vi "TEST_L0_MAJnADDS_NEW.vi"(0 "Instrument VISA in":T1={"AWG VISA"="generadorpulsos", "Oscilloscope  VISA "="Oscilloscope", "Integration Board IP"="172.16.7.43", "connection ID"=refnum, "report out"=refnum, "report file path"=path "C:/Documents and Settings/CTA_LAB01/Desktop/L0_Asic/L0 Asic Test Data"}, 1 "threshold":i32[][](array[numeric])=[[518, 513, 533, 498, 543, 508, 548], [526, 521, 546, 506, 551, 516, 556], [534, 529, 549, 514, 559, 524, 564], [542, 537, 557, 522, 567, 532, 572], [545, 540, 565, 530, 575, 530, 575]], 2 "Serial number":string="SN_023", 11 "error in":errorcluster, 13 "Voltages comprobation":dbl[](array[numeric])=[0.05, 0.1, 0.2, 0.5, 0.8]) -> (4 "Instrument VISA out":T1={"AWG VISA"="generadorpulsos", "Oscilloscope  VISA "="Oscilloscope", "Integration Board IP"="172.16.7.43", "connection ID"=refnum, "report out"=refnum, "report file path"=path "C:/Documents and Settings/CTA_LAB01/Desktop/L0_Asic/L0 Asic Test Data"}, 15 "error out":errorcluster)   [LabVIEW 2009]
uses:
  <vilib>/Utility/NIReport.llb/NI_report.lvclass
  Sum_Abrilader/L0_Sum_Adder Folder/C/Program Files/National Instruments/LabVIEW 2012/instr.lib/Agilent 81150/Agilent 81150.lvlib
  Sum_Abrilader/L0_Sum_Adder Folder/C/Program Files/National Instruments/LabVIEW 2012/instr.lib/Agilent 8000 Series/Agilent 8000 Series.lvlib
panel:
  in  "Attenuation":i32=15
  in  "NChannels":i32[](array[numeric])=[2, 2, 2, 2, 3, 3, 3, 4, 4, 5, 5, 6, 6, 7]
  in  "Channels Combinations":i32[](array[numeric])=[3, 12, 48, 96, 7, 28, 112, 15, 120, 31, 124, 63, 126, 127]
  out "read buffer 4":string="-1.1741E-08;2.232E-09;9.99999E+37;2.976E-09;3.8996E-01;3.7534E-01\n"
  out "ouput data array":dbl[](array[numeric])=[0.2, 127.0, 0.0, 564.0, 0.0, 0.7653, 0.0, 2.976e-09, 0.0, 9.99999e+37, 0.0, 2.232e-09, 0.0, -1.1741e-08, 0.0, 0.0]
  out "read buffer 3":string="V amptd(f2),1.074E+00,0,1.056E+00,1.087E+00,1.0690E+00,5.5E-03,9.4E+01,+ width(f2),2.90015E-09,0,2.90015E-09,2.95960E-09,2.925838E-09,1.2702E-11,9.4E+01,V amptd(1),5.5E-02,0,4.8E-02,6.7E-02,5.55E-02,3.5E-03,9.4E+01,+ width(f1),9.99999E+37,5,9.99999E+37,9.99999E+37,9.99999E+37,9.99999E+37,9.99999E+37,Time(f1-f2),6.26722E-09,0,6.20145E-09,6.35270E-09,6.264189E-09,3.2805E-11,9.4E+01\n"
  in  "Input Voltages":dbl[](array[numeric])=[0.05, 0.2]
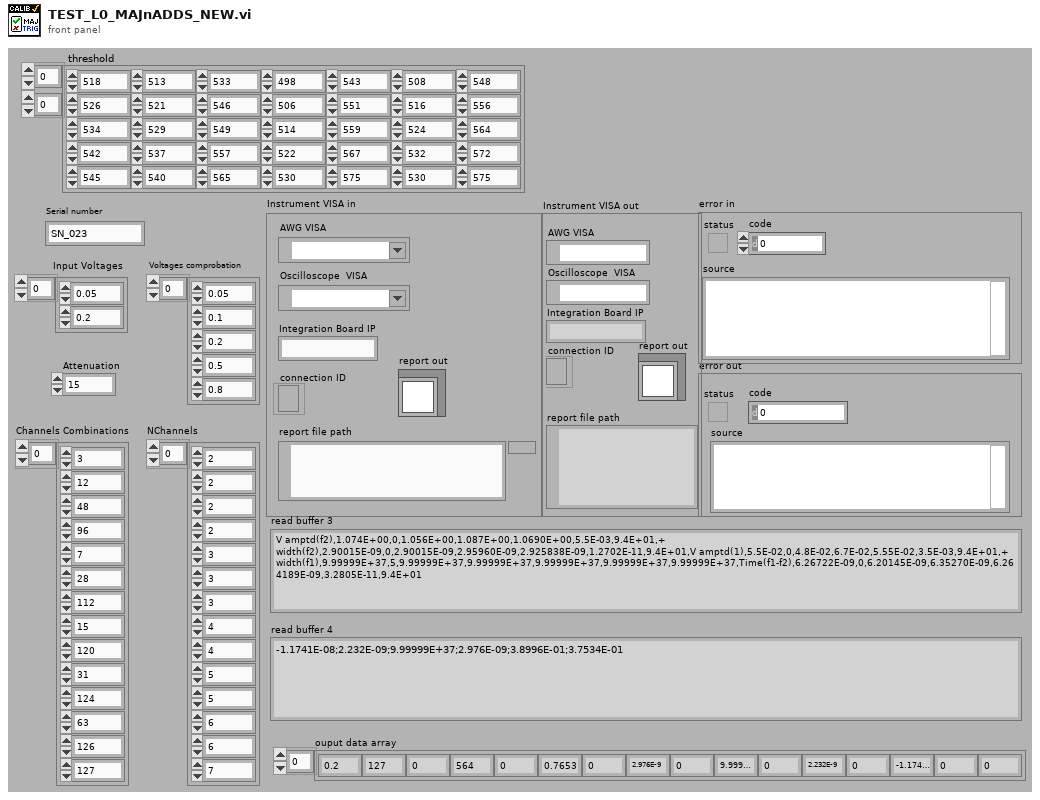
[diagram p1: front panel]
types:
  T1 = cluster{"AWG VISA":refnum<visa-resource-name>, "Oscilloscope  VISA ":refnum<visa-resource-name>, "Integration Board IP":string, "connection ID":refnum<k5>, "report out":refnum<class "NI_report.lvclass">, "report file path":path}
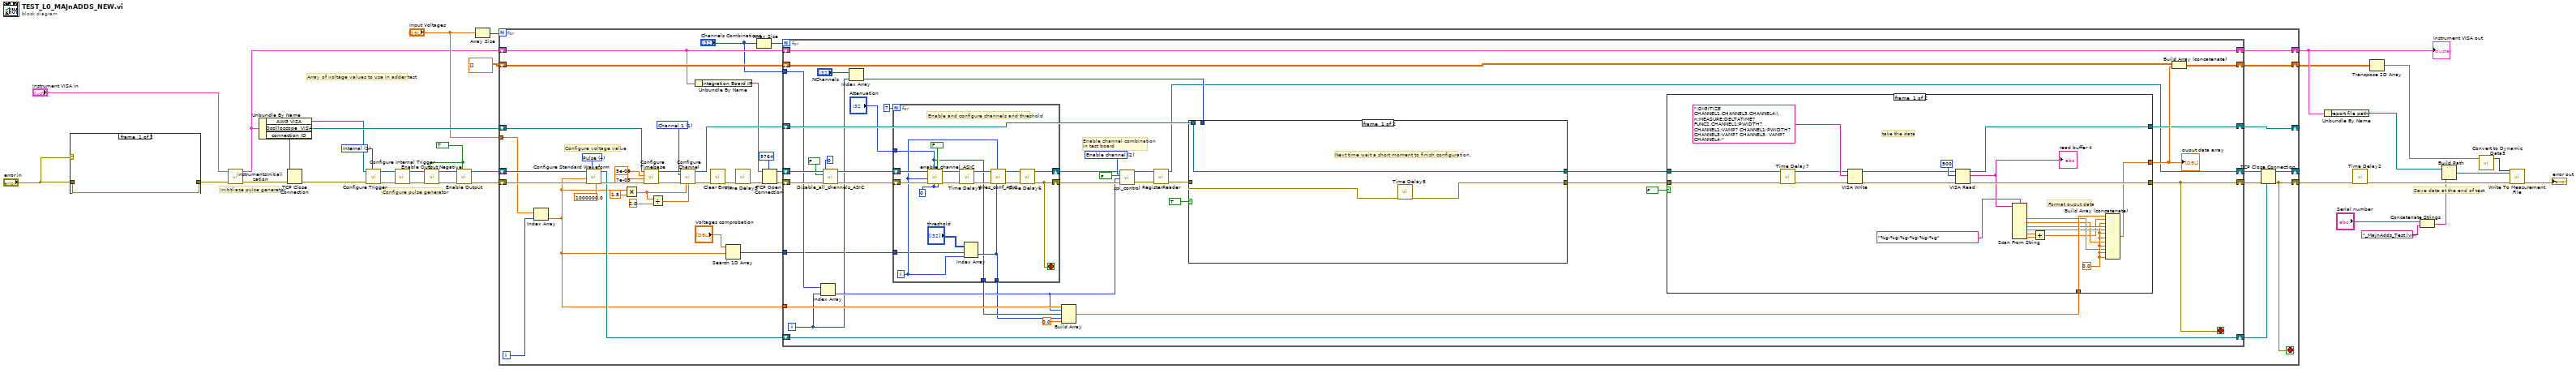
[diagram p0: block diagram]
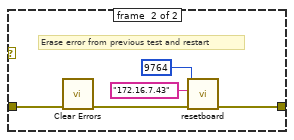
[diagram p2: hidden frame]
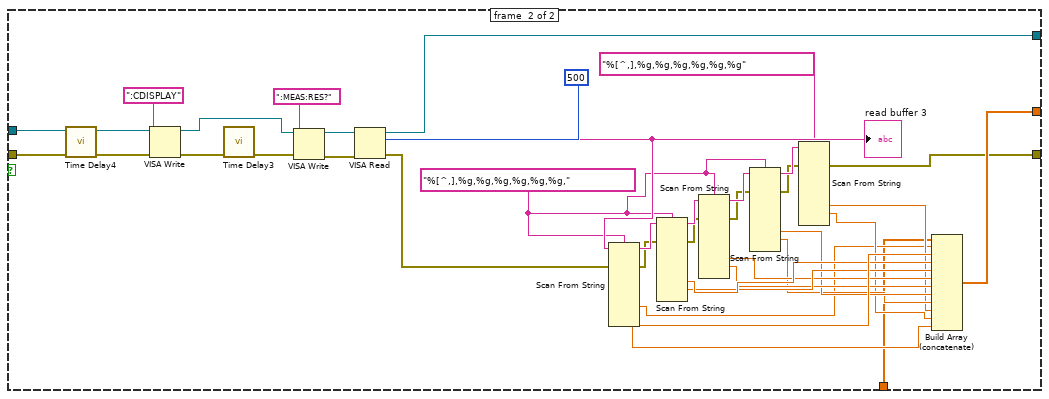
[diagram p3: hidden frame]
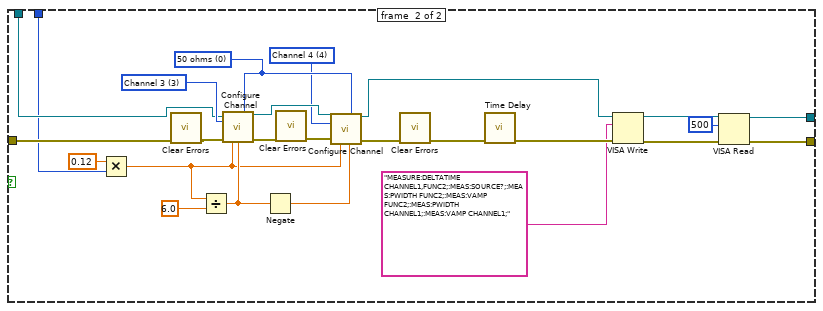
[diagram p4: hidden frame]
diagram:
  w20 = u16 1 items=["Immediate", "Internal", "External", "Software Trigger Function"] ("Trigger Source (0: Immediate)")
  w9 = TRUE ("Enable Output (T: Enable)")
  # "Save data at the end of test"
  # "Array of voltage values to use in adder test"
  # "Configure pulse generator"
  # "Inititliaze pulse generator"
  n1 = case shown="Error" "error in" {
    tunnel: "error in" -> [w35 w37]
    tunnel: [w35 w40] -> w17
    frame #0 {
    }
    frame #1 {
      # "Erase error from previous test and restart"
      n2 = call <vilib>:"Clear Errors.vi"("error in (no error)"=w37) -> ("error out"=w36:errorcluster)  [unwired: 6 in]
      n3 = call "resetboard.vi"("error in (no error)"=w36, "address"="172.16.7.43", "remote port or service name"=u16 9764) -> ("error out"=w40:errorcluster)  [unwired: 7 in, 1 out]
    }
  }
  n4 = call "instrumentsInitialization.vi"("error in"=w17, "Instrument VISA in"="Instrument VISA in") -> ("error out"=w15:errorcluster, "Instrument VISA out"=w4:T1)  [unwired: 8 in]
  n5 = Unbundle By Name(w4) -> ("AWG VISA"=w23:refnum<visa-resource-name>, "Oscilloscope  VISA"=w29:refnum<visa-resource-name>, "connection ID"=w16:refnum<k5>)
  n6 = TCP Close Connection(connection ID=w16, error in (no error)=w15) -> (error out=w1:errorcluster)  [unwired: 1 in, 1 out]
  n7 = call <instrlib>:"Configure Trigger.vi"("Trigger Source (0: Immediate)"=w20, "error in (no error)"=w1, "VISA resource name"=w23) -> ("error out"=w21:errorcluster, "VISA resource name out"=w22:refnum<visa-resource-name>)  [unwired: 7 in]
  n8 = call "Configure Internal Trigger.vi"("error in (no error)"=w21, "VISA resource name"=w22) -> ("error out"=w11:errorcluster, "VISA resource name out"=w12:refnum<visa-resource-name>)  [unwired: 8 in]
  n9 = call "Enable Output Negative.vi"("Enable Output (T: Enable)"=w9, "error in (no error)"=w11, "VISA resource name"=w12) -> ("error out"=w10:errorcluster, "VISA resource name out"=w13:refnum<visa-resource-name>)  [unwired: 7 in]
  n10 = call <instrlib>:"Enable Output.vi"("Enable Output (T: Enable)"=w9, "error in (no error)"=w10, "VISA resource name"=w13) -> ("error out"=w3:errorcluster, "VISA resource name out"=w34:refnum<visa-resource-name>)  [unwired: 7 in]
  n11 = Array Size(array="Input Voltages") -> (size(s)=w30:i32)
  n12 = for {
    N: w30 -> [_]
    shift-right: [w71] -> w24
    shift-left: w3 -> [w80]
    tunnel: "Input Voltages" -> [w78]
    shift-right: [w75] -> w14
    shift-left: w4 -> [w48]
    shift-right: [w74] -> w8
    shift-left: dbl[][] [] -> [w76]
    shift-right: [w72] -> _
    shift-left: w34 -> [w79]
    shift-right: [w73] -> _
    shift-left: w29 -> [w77]
    i -> [w42]
    stop <- w71 stop-if-true
    w62 = 1 items=["Channel 1"=1, "Channel 2"=2, "Channel 3"=3, "Channel 4"=4] ("Channel (1: Channel 1)")
    w70 = u16 4 items=["Sine", "Square", "Ramp Up", "Ramp Down", "Pulse", "Noise", "DC"] ("Waveform (0: Sine)")
    # "Configure voltage value"
    n13 = Index Array(array=w78, index=w42) -> (element=w43:dbl)
    n14 = call <instrlib>:"Configure Standard Waveform.vi"("Frequency (1000.0 Hz)"=1000000.0, "Waveform (0: Sine)"=w70, "error in (no error)"=w80, "Amplitude (1.0 Vpp)"=w43, "VISA resource name"=w79) -> ("error out"=w68:errorcluster, "VISA resource name out"=w51:refnum<visa-resource-name>)  [unwired: 5 in]
    n15 = Multiply(x=w43, y=1.5) -> (x*y=w46:dbl)
    n16 = call "Configure Timebase.vi"("error in (no error)"=w68, "Position (0.0 s)"=7e-09, "Timebase (0.005 s)"=5e-08, "VISA resource name"=w77) -> ("error out"=w67:errorcluster, "VISA resource name out"=w65:refnum<visa-resource-name>)  [unwired: 6 in]
    n17 = Divide(x=w46, y=2.0) -> (x/y=w56:dbl)
    n18 = call "Configure Channel.vi"("VISA resource name"=w65, "Channel (1: Channel 1)"=w62, "error in (no error)"=w67, "Vertical Range (2.0 V)"=w46, "Vertical Offset (0.0 V)"=w56) -> ("VISA resource name out"=w55:refnum<visa-resource-name>, "error out"=w66:errorcluster)  [unwired: 9 in]
    n19 = Unbundle By Name(w48) -> ("Integration Board IP"=w59:string)
    n20 = call <vilib>:"Clear Errors.vi"("error in (no error)"=w66) -> ("error out"=w50:errorcluster)  [unwired: 6 in]
    n21 = Search 1D Array(1D array="Voltages comprobation", element=w43) -> (index of element=w41:i32)  [unwired: 1 in]
    n22 = call "Time Delay5"("error in (no error)"=w50) -> ("error out"=w49:errorcluster)  [unwired: 10 in]
    n23 = Array Size(array="Channels Combinations") -> (size(s)=w45:i32)
    n24 = TCP Open Connection(address=w59, remote port or service name=u16 9764, error in (no error)=w49) -> (connection ID=w52:refnum<k5>, error out=w60:errorcluster)  [unwired: 2 in]
    n25 = for {
      N: w45 -> [_]
      shift-right: [w106] -> w54
      shift-left: w60 -> [w114]
      shift-right: [w115] -> w74
      shift-left: w76 -> [w116]
      shift-right: [w81] -> w53
      shift-left: w52 -> [w105]
      tunnel: w43 -> [w104]
      shift-right: [w101] -> w73
      shift-left: w55 -> [w109]
      shift-right: [w100] -> w72
      shift-left: w51 -> [w100]
      shift-right: [w96] -> w75
      shift-left: w48 -> [w96]
      tunnel: "Channels Combinations" -> [w93]
      tunnel: w41 -> [w86]
      i -> [w89]
      stop <- w106 stop-if-true
      w113 = u16 2 items=["Attenuation", "Clipping", "Enable channel", "Delay line", "ASIC"] ("Device")
      # "Enable channel combination \nin test board"
      n26 = Index Array(array=w93, index=w89) -> (element=w92:i32)
      n27 = call "Disable_all_channels_ASIC.vi"("error in"=w114, "id_in"=0 ("Data"), "Clip_en_b"=FALSE, "connection ID"=w105) -> ("error out"=w118:errorcluster, "connection ID out"=w117:refnum<k5>)  [unwired: 5 in, 1 out]
      n28 = Index Array(array="NChannels", index=w89) -> (element=w88:i32)
      n29 = for {
        N: u32 7 ("Att gain") -> [_]
        shift-right: [w215] -> w111
        shift-left: w118 -> [w221]
        shift-right: [w216] -> w110
        shift-left: w117 -> [w220]
        tunnel: [w207] -> w103
        tunnel: [w210] -> w91
        tunnel: w86 -> [w208]
        tunnel: "Attenuation" -> [w207]
        i -> [w209]
        stop <- w215 stop-if-true
        w218 = u32 0 ("Ib_clipVb")
        # "Enable and configure channels and threshold"
        n30 = call "enable_channel_ASIC.vi"("Clip_sel_b"=w218, "maj/sum"=FALSE, "Ib_clipVb"=w218, "Att gain"=w207, "error in"=w221, "Channel"=w209, "connection ID"=w220) -> ("error out"=w212:errorcluster, "connection ID out"=w217:refnum<k5>)  [unwired: 2 in, 1 out]
        n31 = call "Time Delay9"("error in (no error)"=w212) -> ("error out"=w213:errorcluster)  [unwired: 10 in]
        n32 = Index Array(array="threshold", index (row)=w208, index (col)=w209) -> (element=w210:i32)
        n33 = call "thres_conf_ASIC.vi"("threshold"=w210, "Ring"=w209, "error out 3"=w213, "connection ID"=w217) -> ("error out 2"=w214:errorcluster, "connection ID out"=w216:refnum<k5>)  [unwired: 4 in, 2 out]
        n34 = call "Time Delay6"("error in (no error)"=w214) -> ("error out"=w215:errorcluster)  [unwired: 10 in]
      }
      n35 = Build Array(w104, w92, w103, w91, 0.0 ("element")) -> (w102:dbl[])
      n36 = call "spi_control.vi"("connection ID"=w110, "Device"=w113, "Read/#write"=FALSE, "Data"=w92, "error out 3"=w111) -> ("connection ID out"=w82:refnum<k5>, "error out 2"=w84:errorcluster)  [unwired: 7 in, 6 out]
      n37 = call "RegisterReader.vi"("error in (no error)"=w84, "connection ID"=w82) -> ("error out"=w83:errorcluster, "connection ID out"=w81:refnum<k5>)  [unwired: 7 in]
      n38 = case shown="True" TRUE {
        tunnel: [w179 w192] -> w98
        tunnel: w83 -> [w180 w187]
        tunnel: w109 -> [w181 w188]
        tunnel: [w181 w198] -> w108
        tunnel: w88 -> [_ w183]
        frame #0 {
          # "Next time wait a short moment to finish configuration."
          n39 = call "Time Delay8"("error in (no error)"=w180) -> ("error out"=w179:errorcluster)  [unwired: 10 in]
        }
        frame #1 {
          w199 = u32 0 items=["50 ohms", "1 Mohms"] ("Input Impedance (1: 1 Mohms)")
          w191 = 3 items=["Channel 1"=1, "Channel 2"=2, "Channel 3"=3, "Channel 4"=4] ("Channel (1: Channel 1)")
          w190 = 4 items=["Channel 1"=1, "Channel 2"=2, "Channel 3"=3, "Channel 4"=4] ("Channel (1: Channel 1)")
          n40 = Multiply(x=0.12 ("y"), y=w183) -> (x*y=w184:dbl)
          n41 = call <vilib>:"Clear Errors.vi"("error in (no error)"=w187) -> ("error out"=w205:errorcluster)  [unwired: 6 in]
          n42 = Divide(x=w184, y=6.0) -> (x/y=w185:dbl)
          n43 = call "Configure Channel.vi"("VISA resource name"=w188, "Input Impedance (1: 1 Mohms)"=w199, "Channel (1: Channel 1)"=w191, "error in (no error)"=w205, "Vertical Range (2.0 V)"=w184, "Vertical Offset (0.0 V)"=w185) -> ("VISA resource name out"=w203:refnum<visa-resource-name>, "error out"=w206:errorcluster)  [unwired: 8 in]
          n44 = Negate(x=w185) -> (-x=w189:dbl)
          n45 = call <vilib>:"Clear Errors.vi"("error in (no error)"=w206) -> ("error out"=w197:errorcluster)  [unwired: 6 in]
          n46 = call "Configure Channel.vi"("VISA resource name"=w203, "Input Impedance (1: 1 Mohms)"=w199, "Channel (1: Channel 1)"=w190, "error in (no error)"=w197, "Vertical Range (2.0 V)"=w184, "Vertical Offset (0.0 V)"=w189) -> ("VISA resource name out"=w195:refnum<visa-resource-name>, "error out"=w204:errorcluster)  [unwired: 8 in]
          n47 = call <vilib>:"Clear Errors.vi"("error in (no error)"=w204) -> ("error out"=w196:errorcluster)  [unwired: 6 in]
          n48 = call "Time Delay"("error in (no error)"=w196) -> ("error out"=w194:errorcluster)  [unwired: 10 in]
          n49 = VISA Write(VISA resource name=w195, write buffer="MEASURE:DELTATIME CHANNEL1,FUNC2;:MEAS:SOURCE?;:MEAS:PWIDTH FUNC2;:MEAS:VAMP FUNC2;:MEAS:PWIDTH CHANNEL1;:MEAS:VAMP CHANNEL1;", error in (no error)=w194) -> (VISA resource name out=w202:refnum<visa-resource-name>, error out=w201:errorcluster)  [unwired: 1 out]
          n50 = VISA Read(VISA resource name=w202, byte count=u32 500, error in (no error)=w201) -> (VISA resource name out=w198:refnum<visa-resource-name>, error out=w192:errorcluster)  [unwired: 2 out]
        }
      }
      n51 = case shown="False" FALSE {
        tunnel: w108 -> [w137 w149]
        tunnel: [w132 w147] -> w107
        tunnel: [w135 w146] -> w106
        tunnel: w102 -> [w133 w144]
        tunnel: [w134 w143] -> w101
        tunnel: w98 -> [w136 w141]
        frame #0 {
          w128 = 0.0 ("output 7")
          # "Format ouput data"
          # "take the data"
          n52 = call "Time Delay7"("error in (no error)"=w136) -> ("error out"=w138:errorcluster)  [unwired: 10 in]
          n53 = VISA Write(VISA resource name=w137, write buffer=":DIGITIZE CHANNEL1,CHANNEL3,CHANNEL4;\n:MEASURE:DELTATIME? FUNC2,CHANNEL1;PWIDTH? CHANNEL1;VAMP? CHANNEL1;PWIDTH? CHANNEL3;VAMP? CHANNEL3; VAMP? CHANNEL4;", error in (no error)=w138) -> (VISA resource name out=w131:refnum<visa-resource-name>, error out=w130:errorcluster)  [unwired: 1 out]
          n54 = VISA Read(VISA resource name=w131, byte count=u32 500, error in (no error)=w130) -> (VISA resource name out=w134:refnum<visa-resource-name>, read buffer=w127:string, error out=w135:errorcluster)  [unwired: 1 out]
          "read buffer 4" <- w127
          n55 = Scan From String(format string="%g;%g;%g;%g;%g;%g", input string=w127) -> (output 1=w125:dbl, output 2=w124:dbl, output 3=w129:dbl, output 4=w123:dbl, output 5=w122:dbl, output 6=w121:dbl)  [unwired: 8 in, 3 out]
          n56 = Add(x=w122, y=w121) -> (x+y=w120:dbl)
          n57 = Build Array (concatenate)(w133, w120, w128, w123, w128, w129, w128, w124, w128, w125, w128, w128) -> (w132:dbl[])
        }
        frame #1 {
          w167 = "%[^,],%g,%g,%g,%g,%g,%g," ("format string")
          n58 = call "Time Delay4"("error in (no error)"=w141) -> ("error out"=w142:errorcluster)  [unwired: 10 in]
          n59 = VISA Write(VISA resource name=w149, write buffer=":CDISPLAY", error in (no error)=w142) -> (VISA resource name out=w152:refnum<visa-resource-name>, error out=w150:errorcluster)  [unwired: 1 out]
          n60 = call "Time Delay3"("error in (no error)"=w150) -> ("error out"=w173:errorcluster)  [unwired: 10 in]
          n61 = VISA Write(VISA resource name=w152, write buffer=":MEAS:RES?", error in (no error)=w173) -> (VISA resource name out=w178:refnum<visa-resource-name>, error out=w177:errorcluster)  [unwired: 1 out]
          n62 = VISA Read(VISA resource name=w178, byte count=u32 500, error in (no error)=w177) -> (VISA resource name out=w143:refnum<visa-resource-name>, read buffer=w174:string, error out=w157:errorcluster)  [unwired: 1 out]
          "read buffer 3" <- w174
          n63 = Scan From String(format string=w167, input string=w174, error in=w157) -> (remaining string=w171:string, error out=w153:errorcluster, output 5=w145:dbl, output 6=w172:dbl, output 7=w158:dbl)  [unwired: 12 in, 1 out]
          n64 = Scan From String(format string=w167, input string=w171, error in=w153) -> (remaining string=w168:string, error out=w154:errorcluster, output 5=w165:dbl, output 6=w164:dbl)  [unwired: 13 in, 1 out]
          n65 = Scan From String(format string=w167, input string=w168, error in=w154) -> (remaining string=w169:string, error out=w155:errorcluster, output 5=w163:dbl, output 6=w162:dbl)  [unwired: 13 in, 1 out]
          n66 = Scan From String(format string=w167, input string=w169, error in=w155) -> (remaining string=w170:string, error out=w156:errorcluster, output 5=w161:dbl, output 6=w160:dbl)  [unwired: 13 in, 1 out]
          n67 = Scan From String(format string="%[^,],%g,%g,%g,%g,%g,%g", input string=w170, error in=w156) -> (error out=w146:errorcluster, output 5=w148:dbl, output 6=w159:dbl)  [unwired: 13 in, 2 out]
          n68 = Build Array (concatenate)(w144, w145, w172, w165, w164, w163, w162, w161, w160, w148, w159, w158) -> (w147:dbl[])
        }
      }
      "ouput data array" <- w107
      n69 = Build Array (concatenate)(w116, w107) -> (w115:dbl[][])
    }
    n70 = TCP Close Connection(connection ID=w53, error in (no error)=w54) -> (error out=w71:errorcluster)  [unwired: 1 in, 1 out]
  }
  "Instrument VISA out" <- w14
  n71 = Unbundle By Name(w14) -> ("report file path"=w33:path)
  n72 = call "Time Delay2"("error in (no error)"=w24) -> ("error out"=w31:errorcluster)  [unwired: 10 in]
  n73 = Transpose 2D Array(2D array=w8) -> (transposed array=w18:dbl[][])
  n74 = Concatenate Strings("Serial number", "_MajnAdds_Test.lvm" ("string")) -> (w7:string)
  n75 = Build Path(base path=w33, name or relative path=w7) -> (appended path=w32:path)
  n76 = call "Convert to Dynamic Data3"("2D Array"=w18) -> ("Dynamic Data Type"=w19:dynamicdata)  [unwired: 3 in]
  n77 = call "Write To Measurement File"("Signals"=w19, "error in (no error)"=w31, "Filename"=w32) -> ("error out"=→"error out":errorcluster)  [unwired: 14 in, 2 out]
